vi "Speaker Time Elapsed.vi"(8 "error in":errorcluster, 11 "PAS in":refnum<class "PAS.lvclass">=refnum) -> (0 "error out":errorcluster, 2 "TimeElapsed?":bool, 3 "PAS out":refnum<class "PAS.lvclass">)   [LabVIEW 2014]
uses:
  Switch/Switch.lvclass
  PAS.lvclass
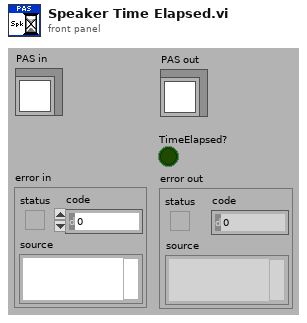
[diagram p1: front panel]
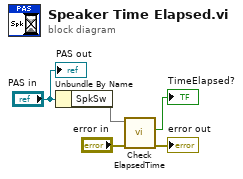
[diagram p0: block diagram]
diagram:
  n1 = Unbundle By Name("PAS in") -> ("SpkSw"=w4)
  n2 = call-dynamic "Check ElapsedTime.vi"("error in"="error in", "Switch in"=w4) -> ("error out"=→"error out":errorcluster, "Cycle Switch?"=→"TimeElapsed?":bool)  [unwired: 6 in, 2 out]
  "PAS out" <- "PAS in"
